vi "IniciarCliente.vi"() -> ()   [LabVIEW 2016]
uses:
  <vilib>/Math Plots/2D Math Plots/2D Error Bar/2D Error Bar XCtrl/2D Error Bar.xctl
  <vilib>/Math Plots/2D Math Plots/2D Error Bar/2D Error Bar Datatype/Public/Plot Helper (Percentage).vi
  <vilib>/Math Plots/2D Math Plots/2D Error Bar/2D Error Bar Datatype/2D Error Bar Datatype.lvclass
panel:
  in  "IP_Servidor":string="localhost"
  in  "Terminar":bool
  in  "Iterações":u32=1000
  in  "Porta_Servidor":u16=3535
  out "size":i32
  out "Resultado":refnum<class "2D Plot Datatype.lvclass">[](xcontrol)
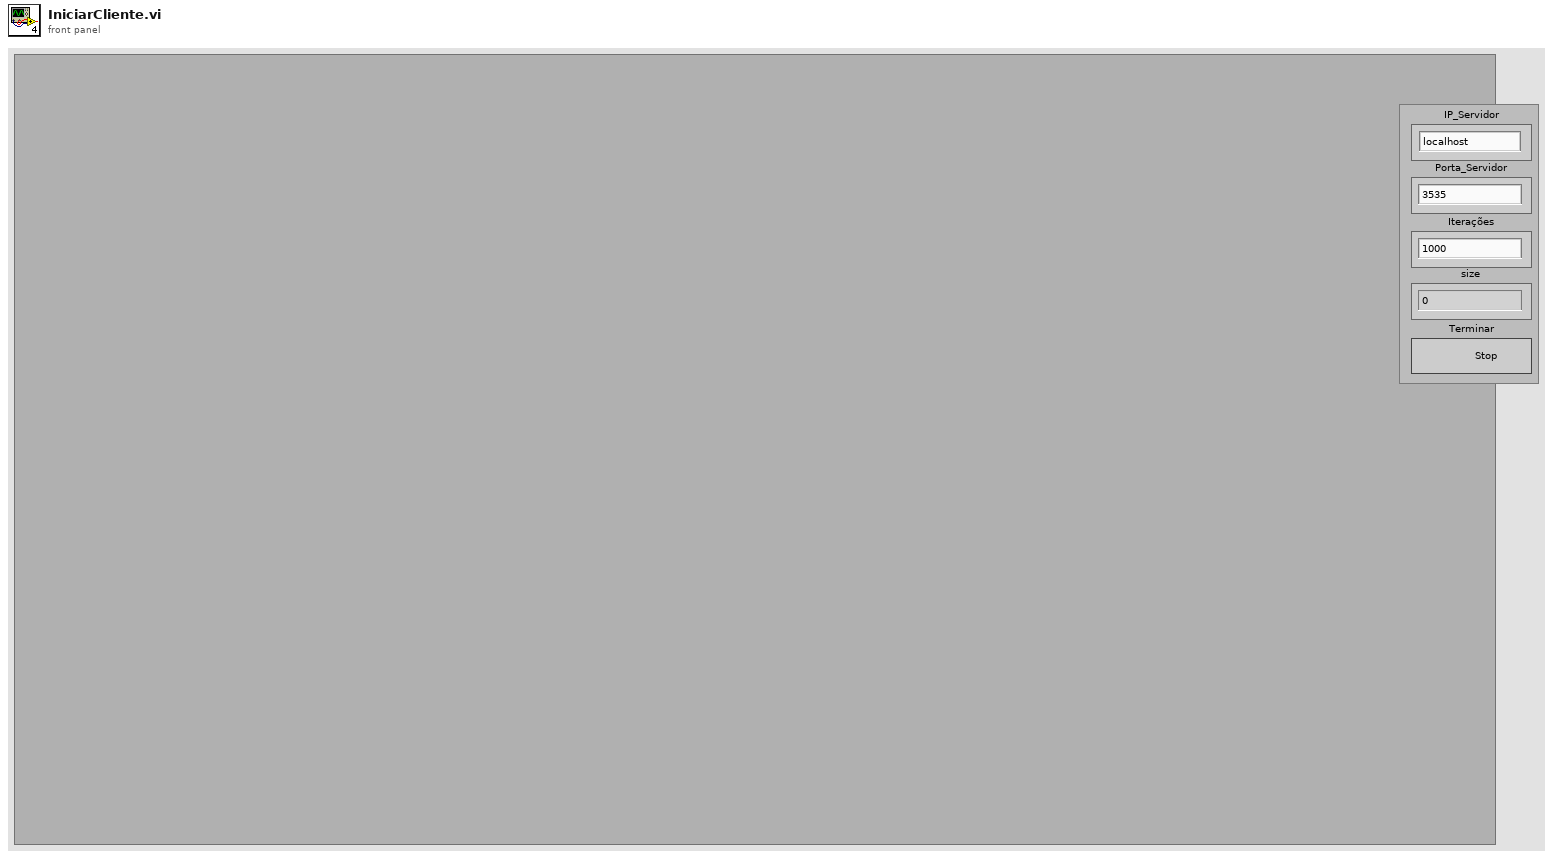
[diagram p1: front panel]
types:
  T1 = enum16{"open", "replace", "create", "open or create", "replace or create", "replace or create with confirmation"}
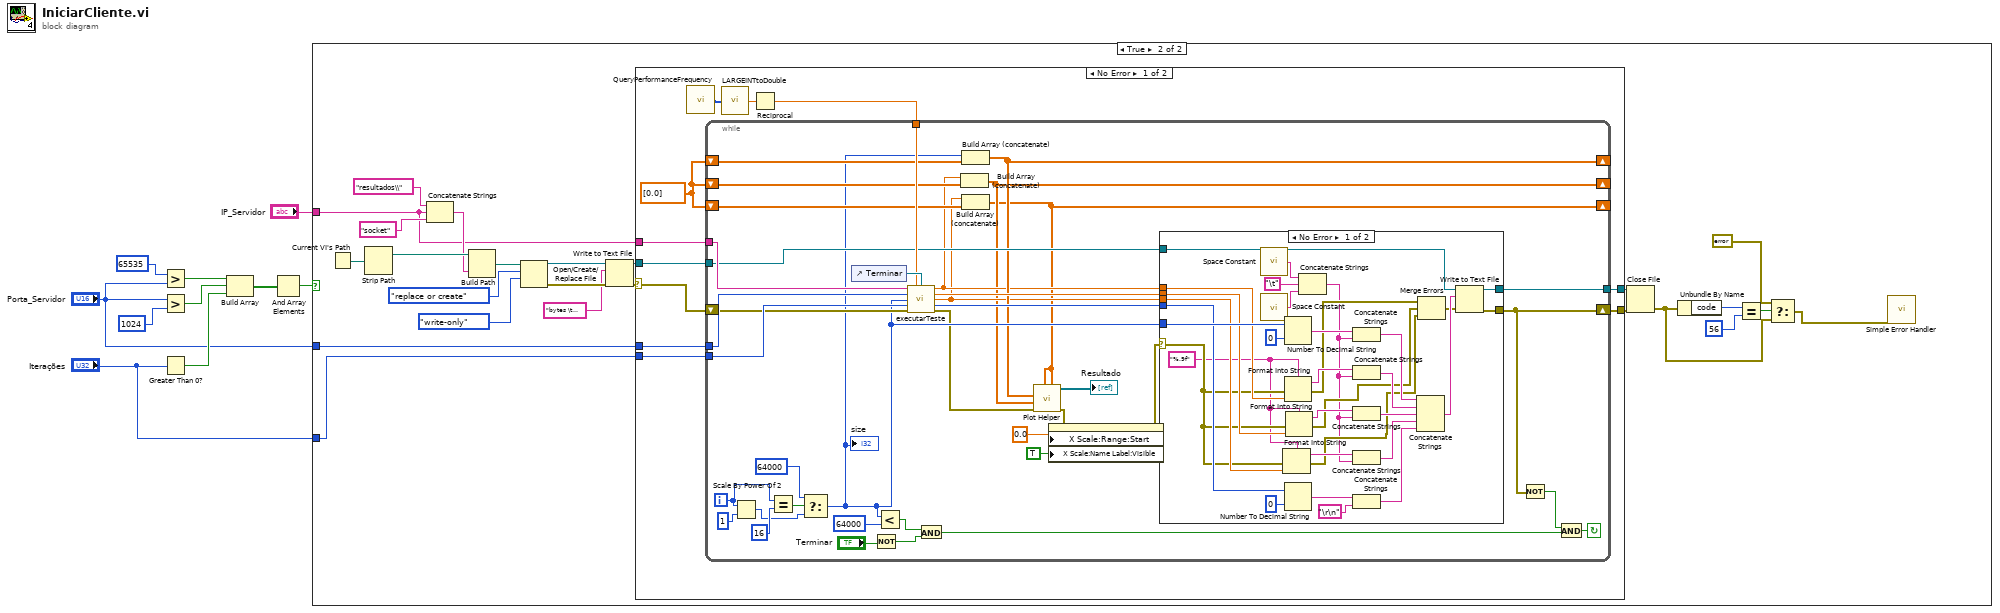
[diagram p0: block diagram]
diagram:
  n1 = Greater?(x=u16 65535, y="Porta_Servidor") -> (0:w7:bool)
  n2 = Greater?(x="Porta_Servidor", y=u16 1024) -> (0:w5:bool)
  n3 = Greater Than 0?(x="Iterações") -> (x > 0?=w6:bool)
  n4 = Build Array(w7, w5, w6) -> (w8:bool[])
  n5 = And Array Elements(Boolean array=w8) -> (logical AND=w4:bool)
  n6 = case shown="True" w4 {
    tunnel: "Iterações" -> [_ w25]
    tunnel: "Porta_Servidor" -> [_ w24]
    tunnel: "IP_Servidor" -> [_ w17]
    frame False {
    }
    frame True {
      n7 = Current VI's Path() -> (path=w22:path)
      n8 = Strip Path(path=w22) -> (stripped path=w21:path)  [unwired: 1 out]
      n9 = Concatenate Strings("resultados\\" ("name or relative path"), w17, "socket" ("string")) -> (w20:string)
      n10 = Build Path(base path=w21, name or relative path=w20) -> (appended path=w33:path)
      n11 = Open/Create/Replace File(file path (use dialog)=w33, operation (0:open)=T1."replace or create", access (0:read/write)=enum16{"read/write", "read-only", "write-only"}."write-only") -> (refnum out=w30:refnum<file>, error out=w29:errorcluster)  [unwired: 3 in, 1 out]
      n12 = Write to Text File(file (use dialog)=w30, text="bytes \t media \t desvio \t erro \t mensagens \n", error in=w29) -> (refnum out=w26:refnum<file>, error out=w28:errorcluster)  [unwired: 1 in, 1 out]
      n13 = case shown="No Error" w28 {
        selector: w28 -> [w37 w120]
        tunnel: [w36 w120] -> w18
        tunnel: [w38 w119] -> w27
        tunnel: w26 -> [w39 w119]
        tunnel: w25 -> [w42 _]
        tunnel: w24 -> [w41 _]
        tunnel: w17 -> [w40 _]
        frame No Error {
          w35 = dbl[] [0.0]
          n14 = call "QueryPerformanceFrequency.vi"() -> ("lpFrequency"=w45:u32[])
          n15 = call "LARGEINTtoDouble.vi"("64Bit Number"=w45) -> ("Double Output"=w44:dbl)
          n16 = Reciprocal(x=w44) -> (1/x=w43:dbl)
          n17 = while {
            tunnel: w43 -> [w76]
            tunnel: w42 -> [w75]
            tunnel: w41 -> [w74]
            tunnel: w40 -> [w73]
            tunnel: w39 -> [w71]
            tunnel: [w72] -> w38
            shift-right: [w66] -> w36
            shift-left: w37 -> [w69]
            shift-right: [w56] -> _
            shift-left: w35 -> [w60]
            shift-right: [w53] -> _
            shift-left: w35 -> [w59]
            shift-right: [w52] -> _
            shift-left: w35 -> [w58]
            i -> [w83]
            stop <- w67 continue-if-true
            n18 = Scale By Power Of 2(n=w83, x=1) -> (x*2^n=w80:i32)
            n19 = Equal?(x=w83, y=16) -> (x = y?=w81:bool)
            n20 = Select(t=64000, s=w81, f=w80) -> (s? t:f=w57:i32)
            "size" <- w57
            n21 = control-ref of="Terminar"() -> (w77:refnum<vi>)
            n22 = Not(x="Terminar") -> (.not. x?=w62:bool)
            n23 = Less?(x=w57, y=64000) -> (x < y?=w63:bool)
            n24 = call "executarTeste.vi"("IP_Servidor"=w73, "frequencia"=w76, "executar?"=w77, "Porta_Servidor"=w74, "tamanho"=w57, "Interações"=w75, "error in (no error)"=w69) -> ("media"=w55:dbl, "desvio"=w70:dbl, "erro"=w54:dbl, "mensagens"=w65:i32, "error out"=w49:errorcluster)  [unwired: 4 in]
            n25 = And(x=w63, y=w62) -> (x .and. y?=w61:bool)
            n26 = Build Array (concatenate)(w55, w59) -> (w53:dbl[])
            n27 = Build Array (concatenate)(w57, w60) -> (w56:dbl[])
            n28 = Build Array (concatenate)(w54, w58) -> (w52:dbl[])
            n29 = call-poly <vilib>:"Plot Helper.vi"("error b percentage"=w52, "error a percentage"=w52, "error in (no error)"=w49, "y vector"=w53, "x vector"=w56) -> ("error out"=w50:errorcluster, "2D Plot Class Obj Array out"=→"Resultado":refnum<class "2D Plot Datatype.lvclass">[])  [unwired: 1 in, 4 out]
            n30 = property on="Resultado" class="2D Error Bar (strict)"(error in=w50, "X Scale:Range:Start"=0.0 ("Y Scale:Range:Minimum"), "X Scale:Name Label:Visible"=TRUE) -> (error out=w48:errorcluster)  [unwired: 1 in, 1 out]
            n31 = case shown="No Error" w48 {
              selector: w48 -> [w86 w118]
              tunnel: [w116 w118] -> w66
              tunnel: [w115 w117] -> w72
              tunnel: w71 -> [w114 w117]
              tunnel: w57 -> [w102 _]
              tunnel: w65 -> [w101 _]
              tunnel: w55 -> [w99 _]
              tunnel: w70 -> [w96 _]
              tunnel: w54 -> [w95 _]
              frame No Error {
                w85 = "%.9f" ("format string")
                n32 = call <vilib>:"Space Constant.vi"() -> ("String"=w88:string)
                n33 = call <vilib>:"Space Constant.vi"() -> ("String"=w90:string)
                n34 = Format Into String(format string=w85, error in=w86, w95) -> (resulting string=w97:string, error out=w91:errorcluster)  [unwired: 1 in]
                n35 = Number To Decimal String(number=w102, width (-)=i16 0) -> (decimal integer string=w111:string)
                n36 = Format Into String(format string=w85, error in=w86, w99) -> (resulting string=w100:string, error out=w94:errorcluster)  [unwired: 1 in]
                n37 = Number To Decimal String(number=w101, width (-)=i16 0) -> (decimal integer string=w113:string)
                n38 = Format Into String(format string=w85, error in=w86, w96) -> (resulting string=w98:string, error out=w92:errorcluster)  [unwired: 1 in]
                n39 = Concatenate Strings(w88, "\t", w90) -> (w87:string)
                n40 = Concatenate Strings(w111, w87) -> (w108:string)
                n41 = Concatenate Strings(w100, w87) -> (w107:string)
                n42 = Concatenate Strings(w98, w87) -> (w106:string)
                n43 = Concatenate Strings(w97, w87) -> (w105:string)
                n44 = Concatenate Strings(w113, "\r\n") -> (w104:string)
                n45 = Concatenate Strings(w108, w107, w106, w105, w104) -> (w103:string)
                n46 = Merge Errors(w94, w92, w91) -> (w93:errorcluster)
                n47 = Write to Text File(file (use dialog)=w114, text=w103, error in=w93) -> (refnum out=w115:refnum<file>, error out=w116:errorcluster)  [unwired: 1 in, 1 out]
              }
              frame Error {
              }
            }
            n48 = Not(x=w66) -> (.not. x?=w68:bool)
            n49 = And(x=w68, y=w61) -> (x .and. y?=w67:bool)
          }
        }
        frame Error {
        }
      }
      n50 = Close File(refnum=w27, error in=w18) -> (error out=w16:errorcluster)  [unwired: 1 out]
      n51 = Unbundle By Name(w16) -> ("code"=w12:i32)
      n52 = Equal?(x=w12, y=56) -> (x = y?=w13:bool)
      n53 = Select(t=errorcluster {"status"=TRUE, "code"=56, "source"="Timeout "}, s=w13, f=w16) -> (s? t:f=w14:errorcluster)
      n54 = call <vilib>:"Simple Error Handler.vi"("error in (no error)"=w14) -> ()  [unwired: 4 in, 5 out]
    }
  }
